vi "DescriptorToVariant.vi"(10 "Descriptor":T1) -> (2 "Variant":variant)   [LabVIEW 2013, in "OpenDescriptor.lvlib"]
uses:
  OpenDescriptor.lvlib
  OpenDescriptor -- cluster.ctl
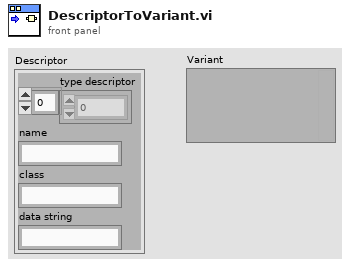
[diagram p1: front panel]
types:
  T1 = typedef "OpenDescriptor.lvlib/OpenDescriptor -- cluster.ctl" = cluster{"type descriptor":i16[], "name":string, "class":string, "data string":string}
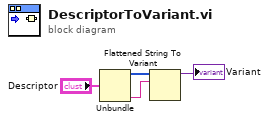
[diagram p0: block diagram]
diagram:
  n1 = Unbundle("Descriptor") -> ("type descriptor"=w4:i16[], "data string"=w3:string)  [unwired: 2 out]
  n2 = Flattened String To Variant(6:w3, 7:w4) -> (3:→"Variant":variant)  [unwired: 1 in, 1 out]
